vi "Get Measurements.vi"(8 "error in (no error)":errorcluster, 11 "SPECAN_IQSLOT in":refnum<class "SPECAN_IQSLOT.lvclass">) -> (0 "error out":errorcluster, 3 "SPECAN_IQSLOT out":refnum<class "SPECAN_IQSLOT.lvclass">)   [LabVIEW 2018, in "SPECAN_IQSLOT.lvlib" / "SPECAN_IQSLOT.lvclass"]
uses:
  SPECAN_IQSLOT.lvclass
  C:/Sequence Automation/Plugins/Measurement Interface.lvlibp/Measurement Interface.lvclass
  Plugins/Measurement Interface.lvlibp/Private Methods/Measurement Parameters/Read Measurement Parameters.vi
  Plugins/String Database.lvlibp/String Database.lvclass
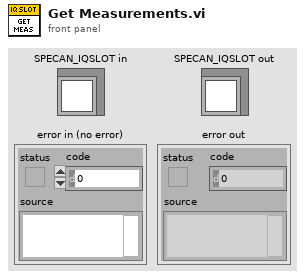
[diagram p1: front panel]
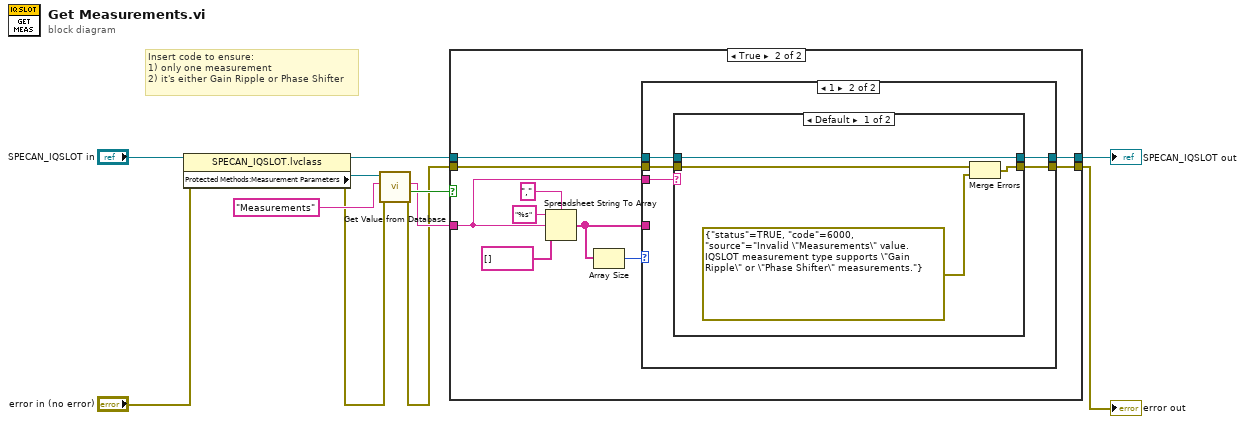
[diagram p0: block diagram]
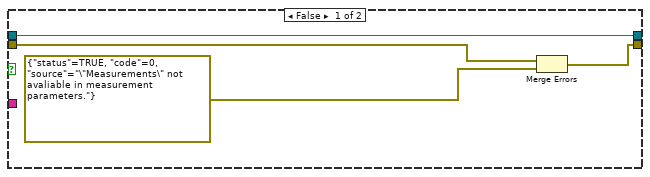
[diagram p2: hidden frame]
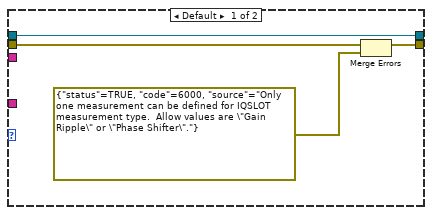
[diagram p3: hidden frame]
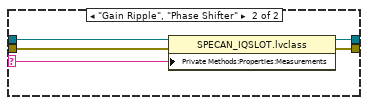
[diagram p4: hidden frame]
diagram:
  # "Insert code to ensure:\n1) only one measurement\n2) it's either Gain Ripple or Phase Shifter"
  n1 = property class="SPECAN_IQSLOT.lvclass"(reference="SPECAN_IQSLOT in", error in="error in (no error)") -> (reference out=w5:refnum<class "SPECAN_IQSLOT.lvclass">, error out=w9:errorcluster, "Protected Methods:Measurement Parameters"=w11:refnum<class "String Database.lvclass">)
  n2 = call "Get Value from Database.vi"("error in (no error)"=w9, "Entry Name"="Measurements", "Message in"=w11) -> ("error out"=w3:errorcluster, "Entry Found"=w8:bool, "Entry Value"=w4:string)  [unwired: 5 in, 1 out]
  n3 = case shown="True" w8 {
    tunnel: w5 -> [w15 w25]
    tunnel: w4 -> [_ w16]
    tunnel: w3 -> [w13 w24]
    tunnel: [w15 w23] -> w2
    tunnel: [w12 w22] -> w1
    frame False {
      n4 = Merge Errors(w13, errorcluster {"status"=TRUE, "code"=0, "source"="\"Measurements\" not avaliable in measurement parameters."} ("error out")) -> (w12:errorcluster)
    }
    frame True {
      n5 = Spreadsheet String To Array(delimiter (Tab)=",", format string="%s", spreadsheet string=w16, array type (2D Dbl)=string[] []) -> (array=w18:string[])
      n6 = Array Size(array=w18) -> (size(s)=w17:i32)
      n7 = case shown="1" w17 {
        tunnel: w25 -> [w29 w34]
        tunnel: w24 -> [w28 w33]
        tunnel: [w29 w32] -> w23
        tunnel: [w27 w31] -> w22
        tunnel: w18 -> [_ _]
        tunnel: w16 -> [_ w30]
        frame Default {
          n8 = Merge Errors(w28, errorcluster {"status"=TRUE, "code"=6000, "source"="Only one measurement can be defined for IQSLOT measurement type.  Allow values are \"Gain Ripple\" or \"Phase Shifter\"."} ("error constant")) -> (w27:errorcluster)
        }
        frame 1 {
          n9 = case shown="Default" w30 {
            selector: w30 -> [_ w39]
            tunnel: w34 -> [w38 w43]
            tunnel: w33 -> [w37 w42]
            tunnel: [w38 w41] -> w32
            tunnel: [w36 w40] -> w31
            frame Default {
              n10 = Merge Errors(w37, errorcluster {"status"=TRUE, "code"=6000, "source"="Invalid \"Measurements\" value.  IQSLOT measurement type supports \"Gain Ripple\" or \"Phase Shifter\" measurements."} ("error constant")) -> (w36:errorcluster)
            }
            frame "Gain Ripple", "Phase Shifter" {
              n11 = property class="SPECAN_IQSLOT.lvclass"(reference=w43, error in=w42, "Private Methods:Properties:Measurements"=w39) -> (reference out=w41:refnum<class "SPECAN_IQSLOT.lvclass">, error out=w40:errorcluster)
            }
          }
        }
      }
    }
  }
  "error out" <- w1
  "SPECAN_IQSLOT out" <- w2
